vi "main OP600_V2 (AUTOMATISATION).vi"() -> ()   [LabVIEW 2020]
uses:
  Lib/02 SLIM ZEN WS 500/SubVi/FGV.ctl
  SubVI/CheminDeBase.vi
  SubVI/OP500ZP_state.ctl
  VG/VG_progressBar.vi
  VG/IS30%.vi
  VG/PN.vi
  VG/PackType.vi
  SubVI/OP500ZP_VGConf.vi
  VG/Ubatt.vi
panel:
  out "IS30% ?":bool
  out "Cluster":T1
  out "VISA OUT":T2
  out "progression":u8(slide) scale=0.0..100.0
  out "PN":string
  out "errout 2":errorcluster={"status"=TRUE, "code"=0, "source"="PCAN_CHANNEL ILLEGAL"} caption="errout"
  out "errout":errorcluster caption="sortie d'erreur"
  out "STOP":bool
  out "TOP":string
  out "DRAW":picture
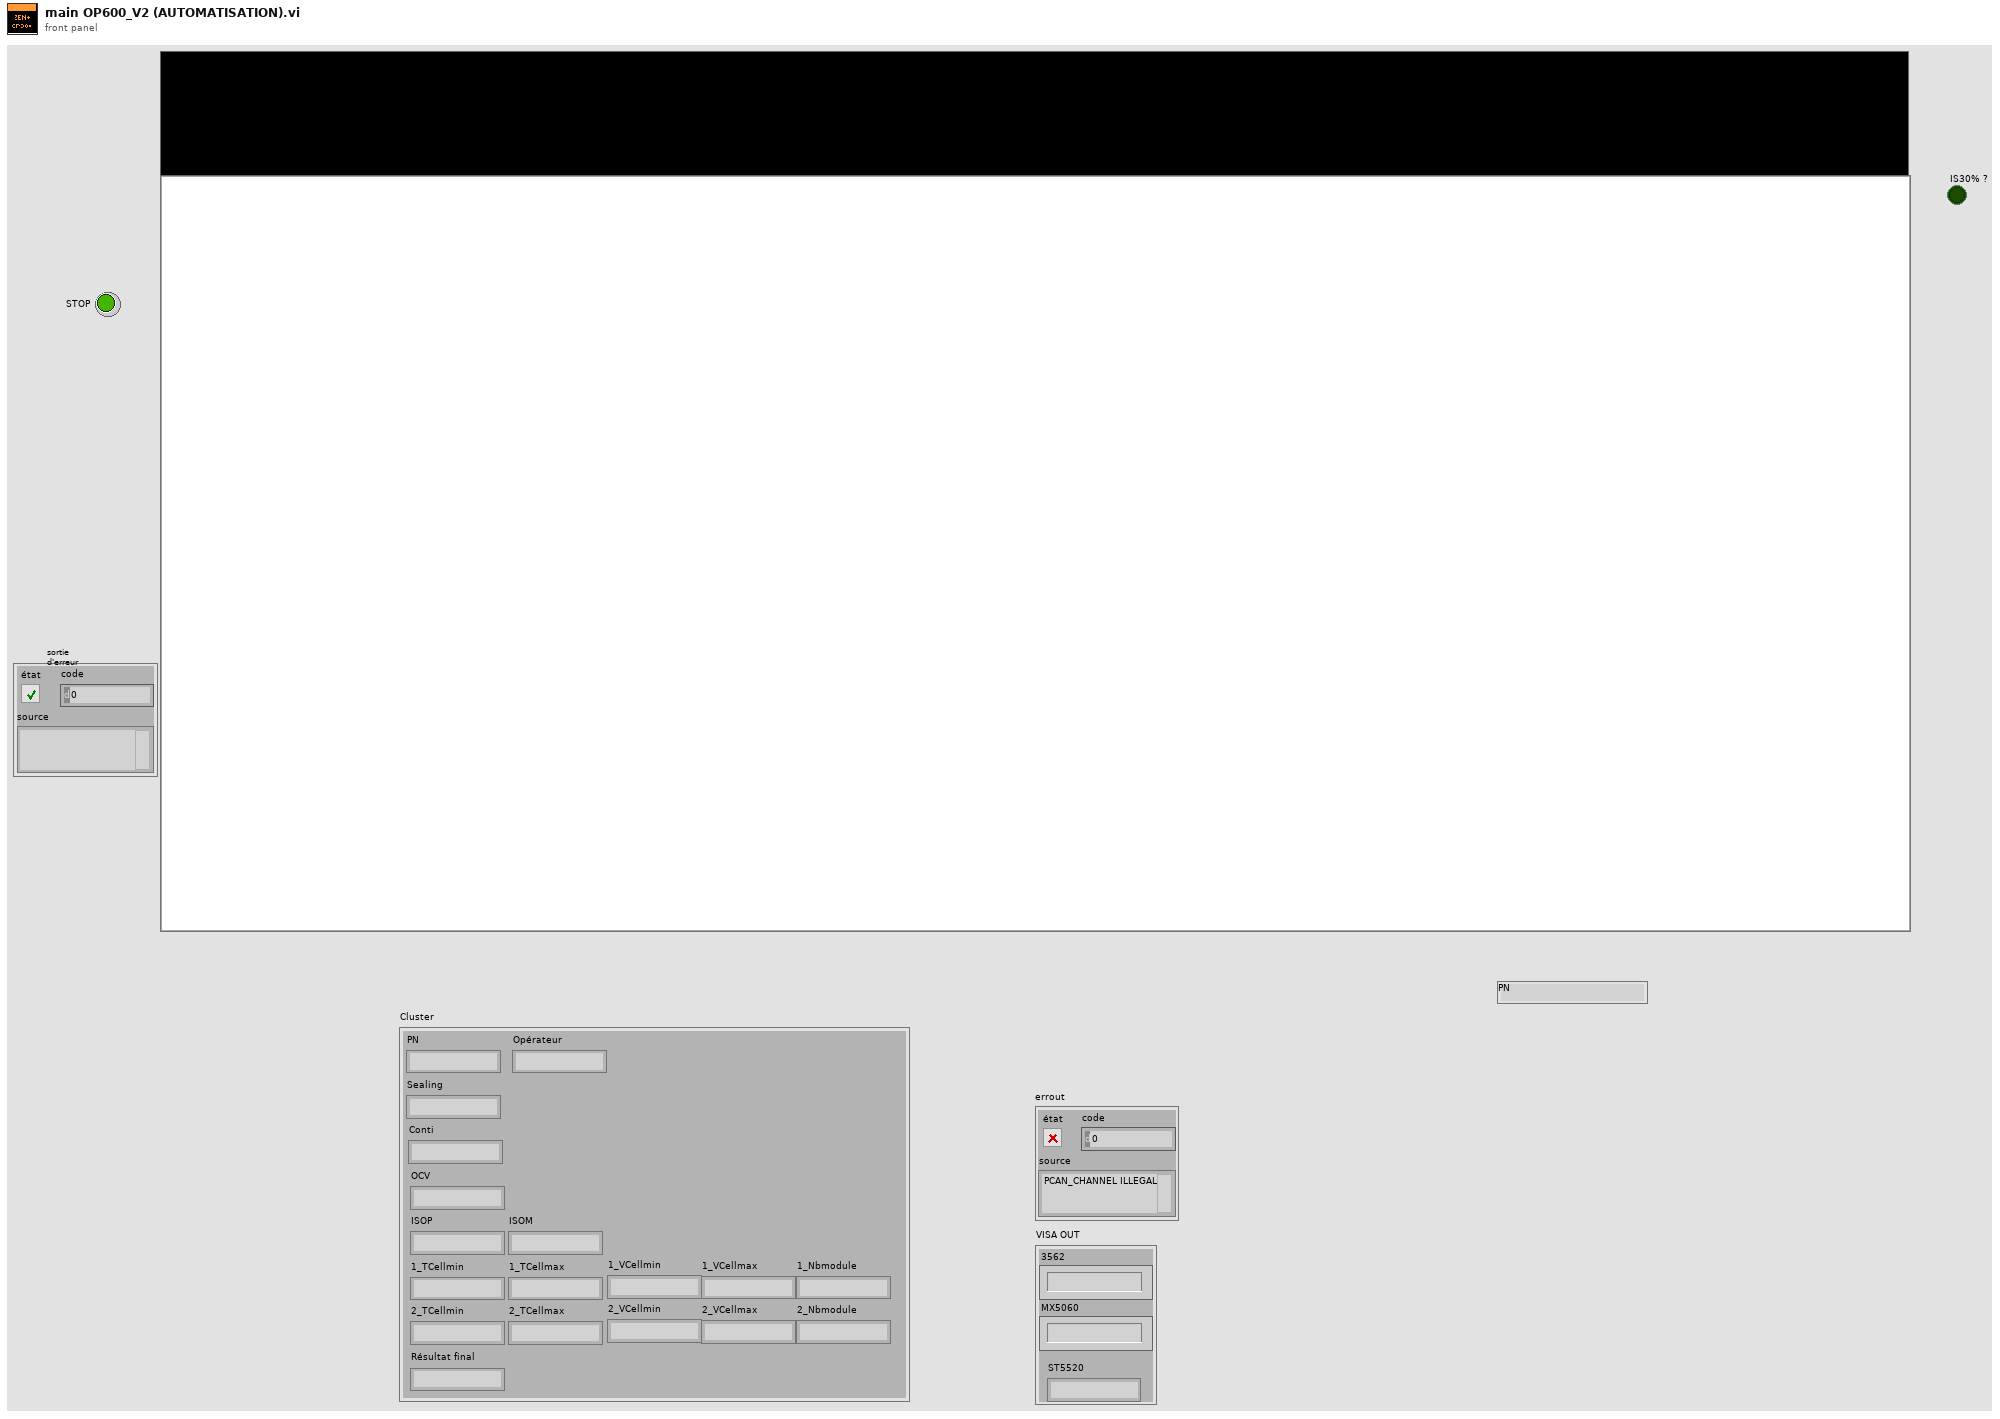
[diagram p1: front panel]
types:
  T1 = cluster{"PN":string, "Opérateur":string, "Sealing":string, "Conti":string, "OCV":string, "ISOP":string, "ISOM":string, "1_TCellmin":string, "1_TCellmax":string, "1_VCellmin":string, "1_VCellmax":string, "1_Nbmodule":string, "2_TCellmin":string, "2_TCellmax":string, "2_VCellmin":string, "2_VCellmax":string, "2_Nbmodule":string, "Résultat final":string}
  T2 = cluster{"3562":string, "MX5060":string, "ST5520":string}
  T3 = cluster{"PN":string, "Sealing":string, "Opérateur":string, "Conti":string, "OCV":string, "ISOP":string, "ISOM":string, "1_TCellmin":string, "1_TCellmax":string, "1_VCellmin":string, "1_VCellmax":string, "1_Nbmodule":string, "2_TCellmin":string, "2_TCellmax":string, "2_VCellmin":string, "2_VCellmax":string, "2_Nbmodule":string, "Résultat final":string}
  T4 = typedef "OP500ZP_state.ctl" = enum16{"Null", "Demarrage", "Init", "Scan", "Iso", "Softs", "MCU", "OCVACIR", "Conti", "DTC", "DataDyn", "DataDyn2", "Crash", "Next", "Comext"}
  T5 = typedef "FGV.ctl" = enum16{"GET", "SET", "RAZ"}
  T6 = typedef "OP500ZP_state.ctl" = enum16{"Null", "Demarrage", "Init", "Scan", "Montage", "Conti", "OCV", "Iso", "Softs", "Vpack", "DataDyn", "Dessouter", "DataDyn2", "Demontage", "Crash", "Next", "Sealing", "Comext"}
  T7 = cluster{"Chaîne":string, "Chaîne":string, "Chaîne":string, "Chaîne":string, "Chaîne":string, "Chaîne":string, "Chaîne":string, "Chaîne 2":string}
  T8 = typedef "imagedata.ctl" = cluster{"image type":i32, "image depth":i32, "image":u8[], "mask":u8[], "colors":u32[], "Rectangle":cluster{"left":i16, "top":i16, "right":i16, "bottom":i16}}
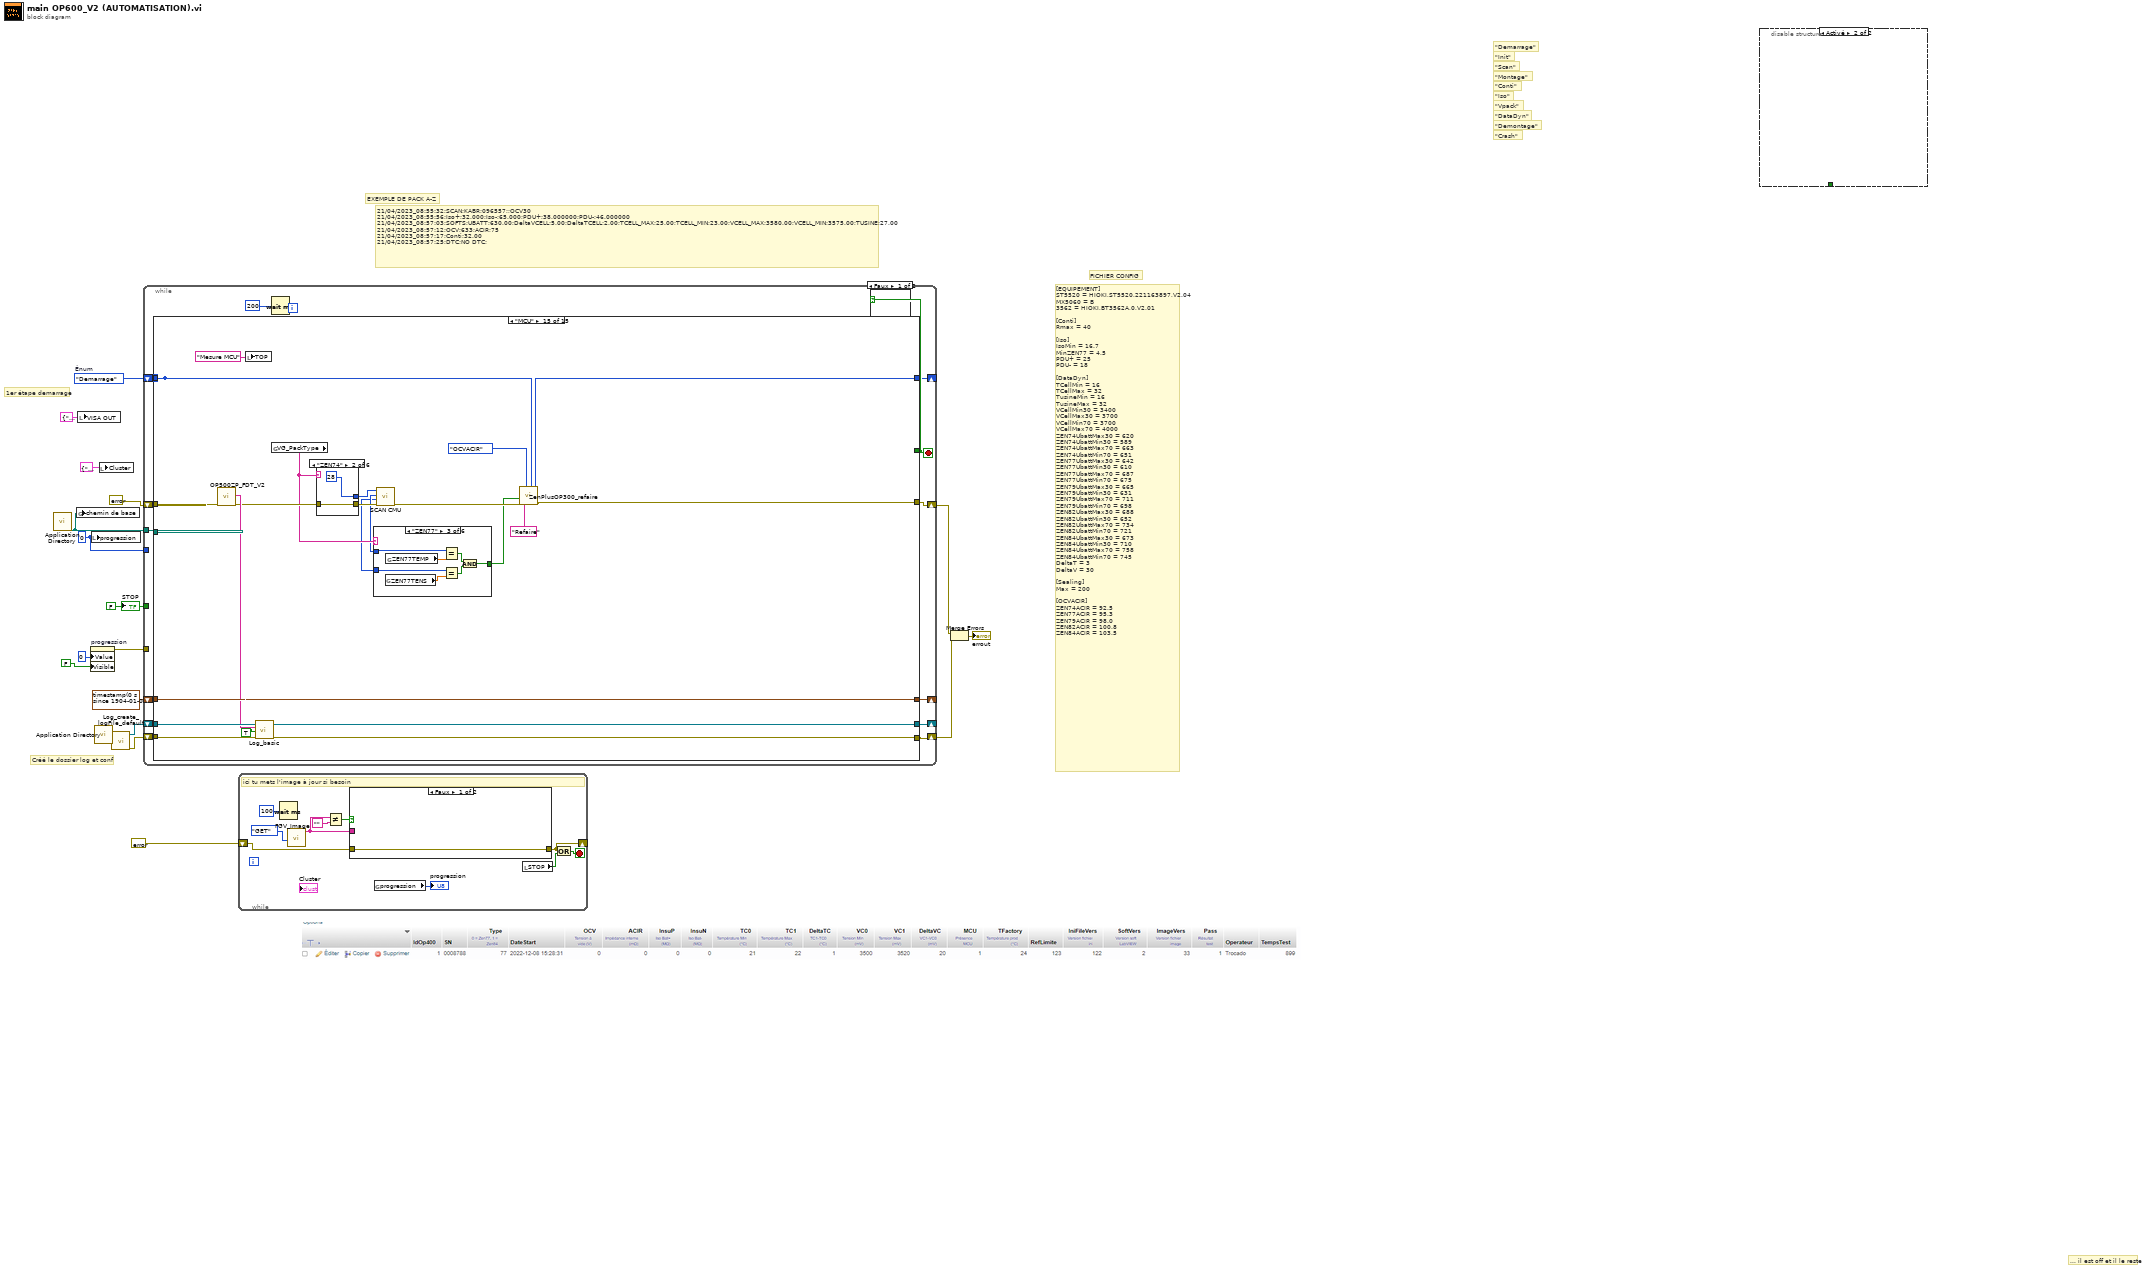
[diagram p0: block diagram]
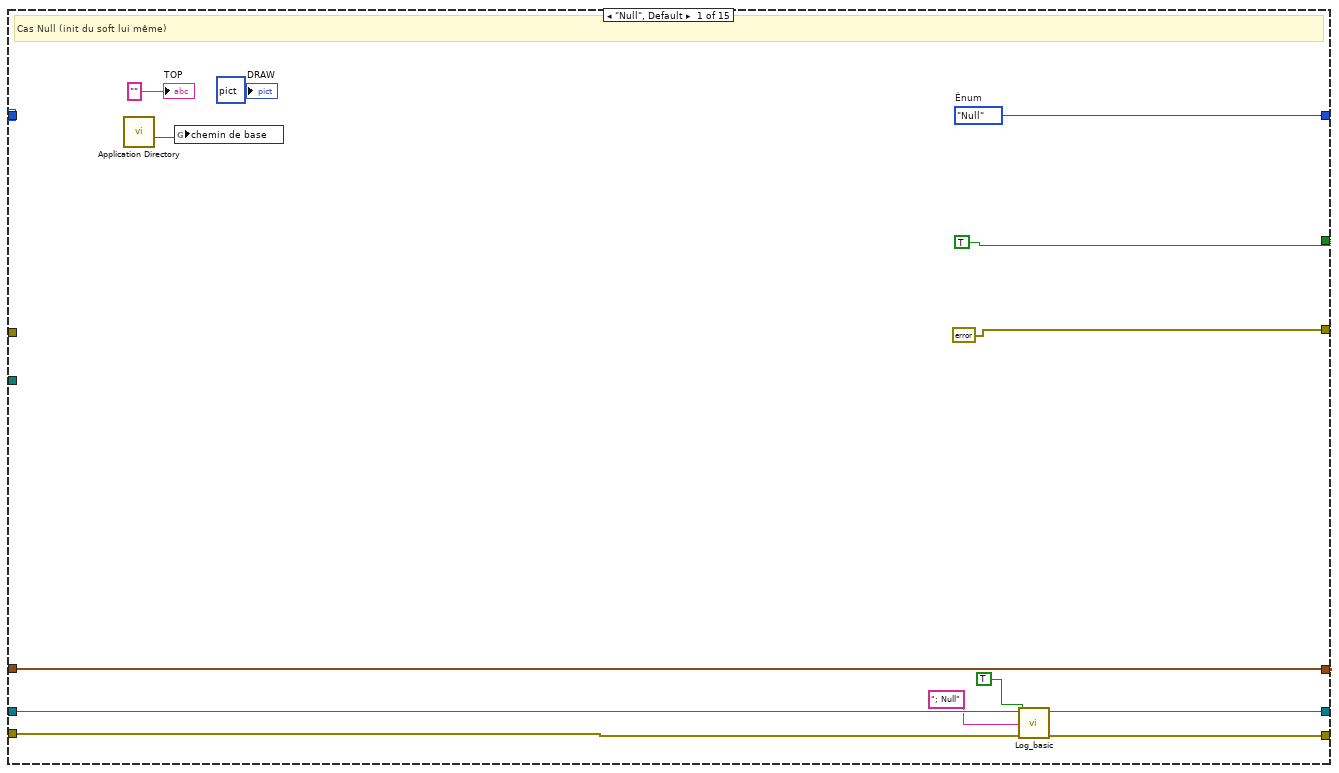
[diagram p2: hidden frame]
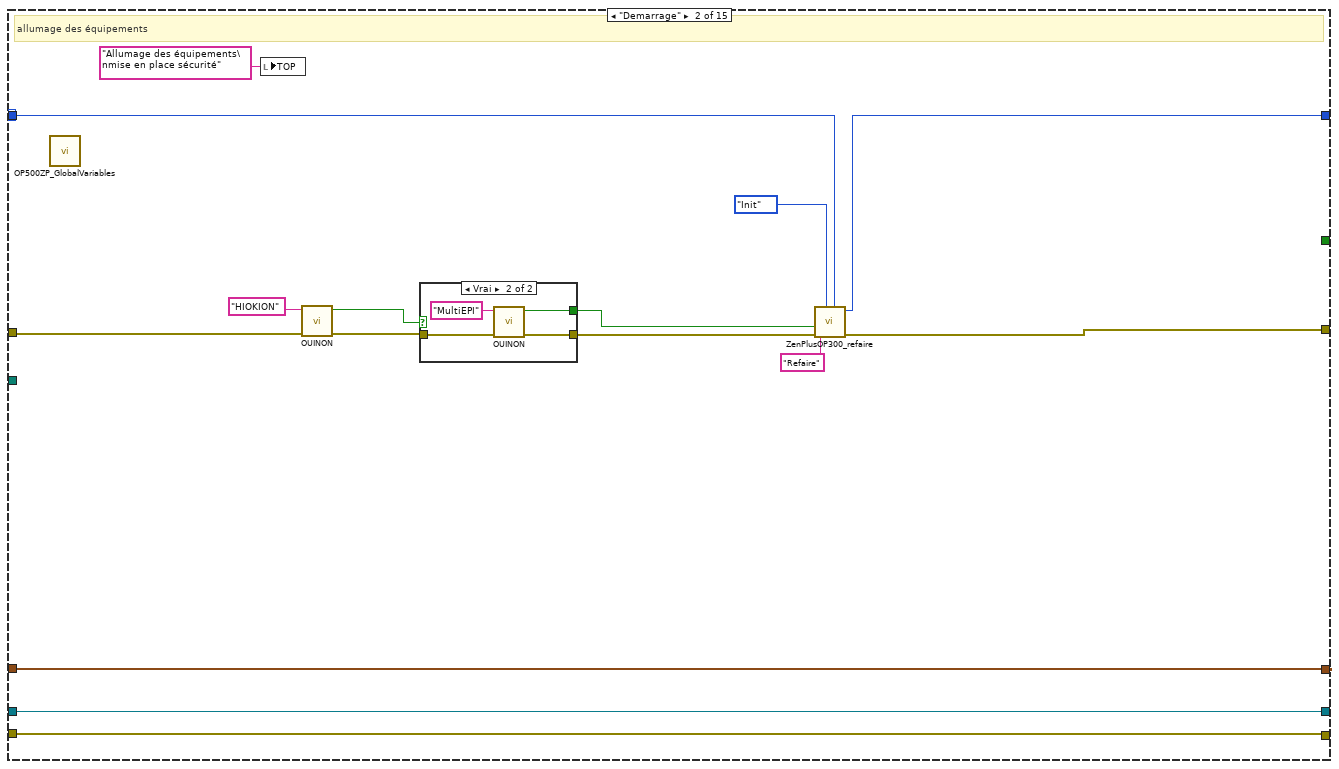
[diagram p3: hidden frame]
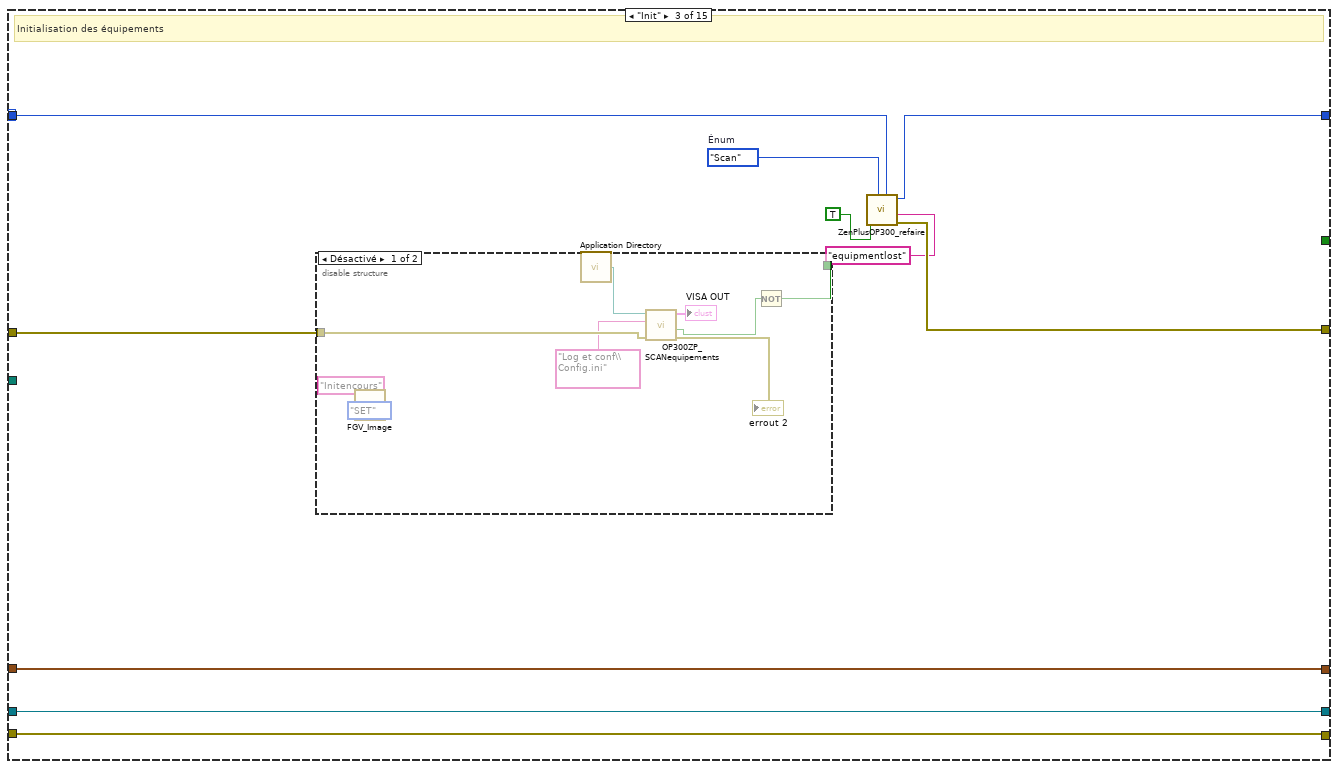
[diagram p5: hidden frame]
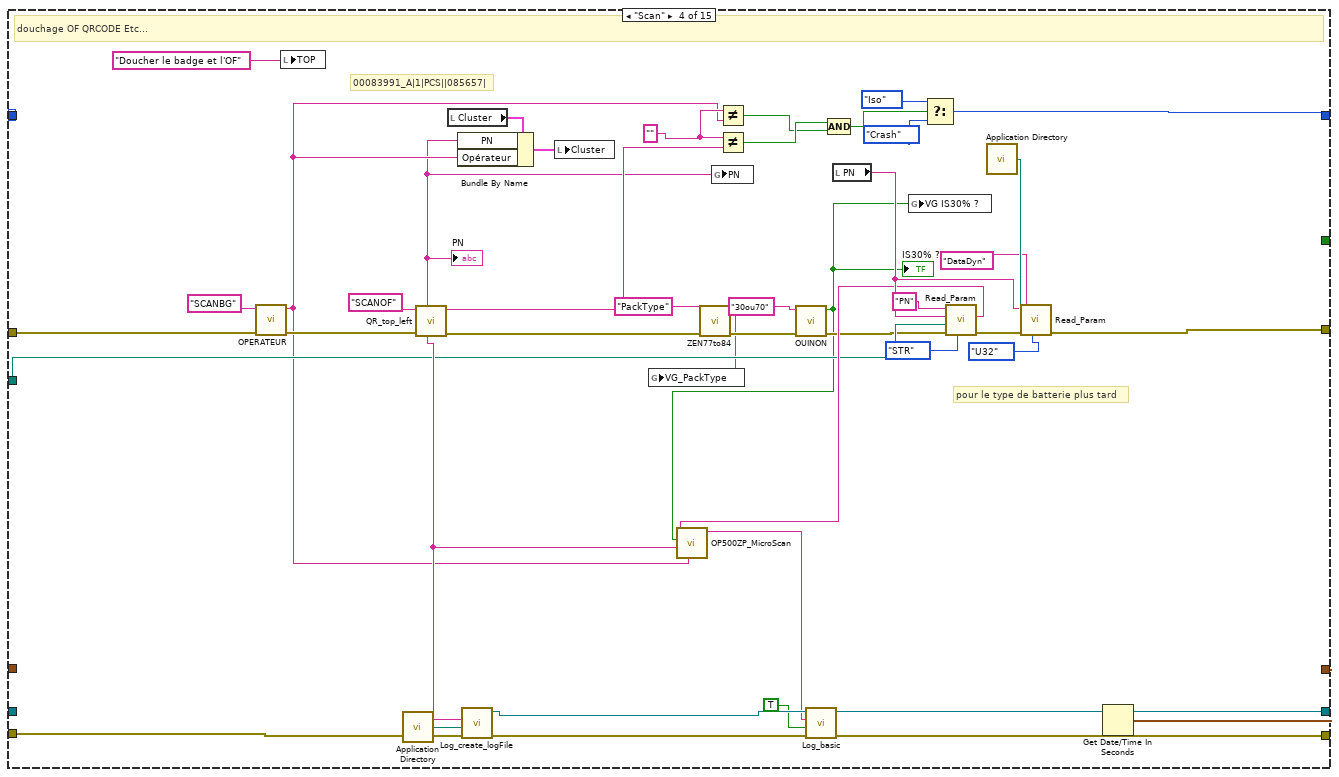
[diagram p7: hidden frame]
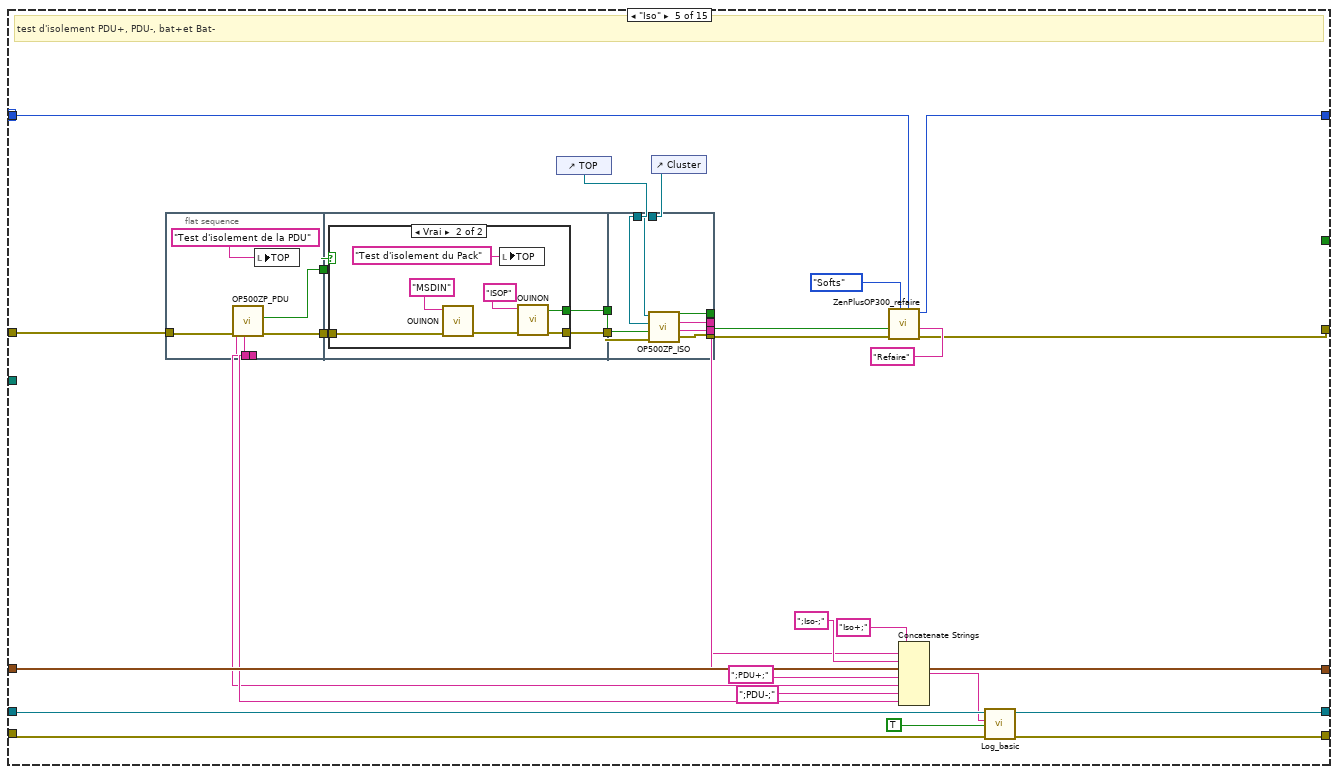
[diagram p8: hidden frame]
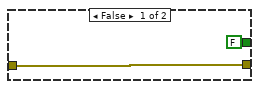
[diagram p9: hidden frame]
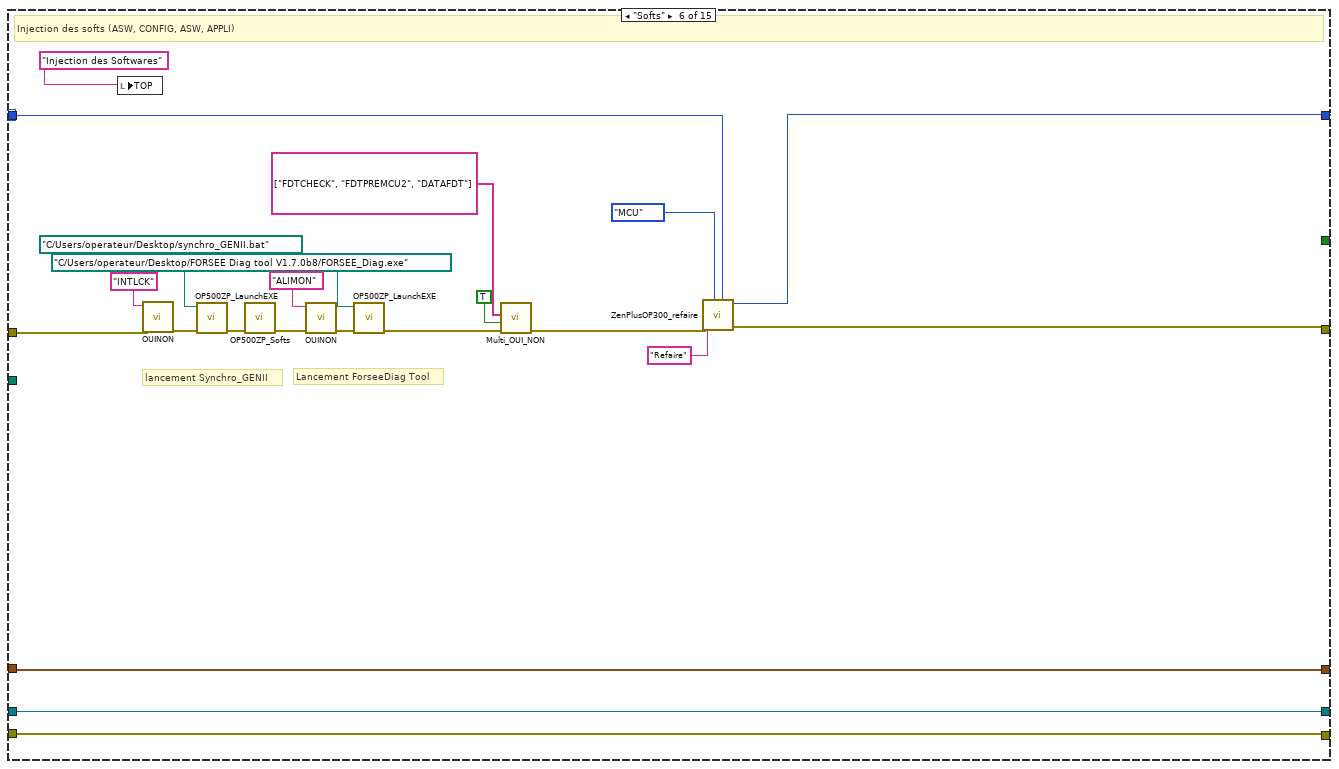
[diagram p10: hidden frame]
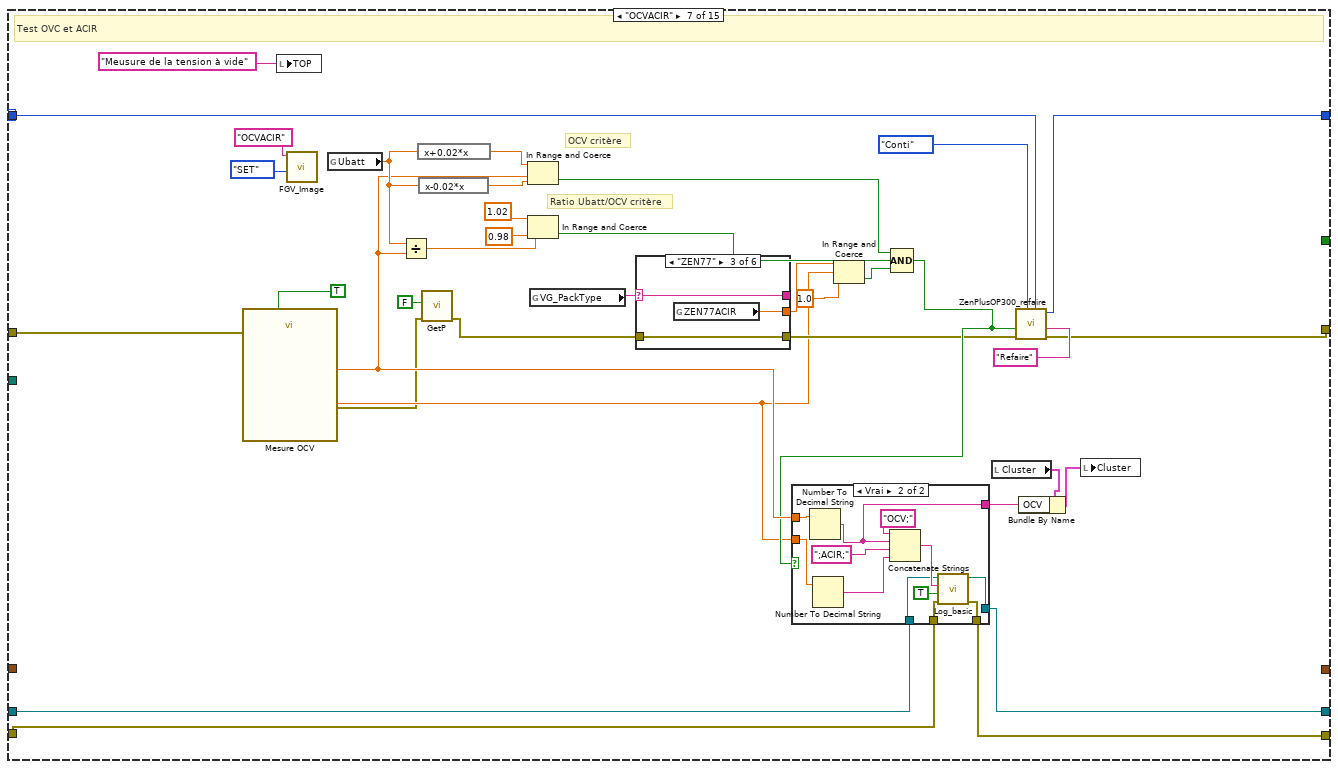
[diagram p11: hidden frame]
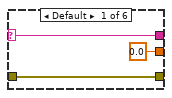
[diagram p12: hidden frame]
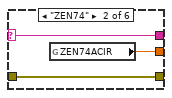
[diagram p13: hidden frame]
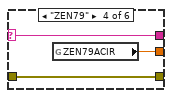
[diagram p14: hidden frame]
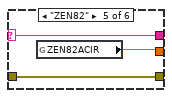
[diagram p15: hidden frame]
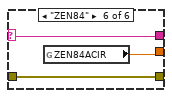
[diagram p16: hidden frame]
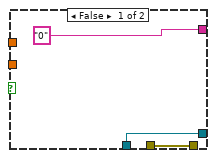
[diagram p17: hidden frame]
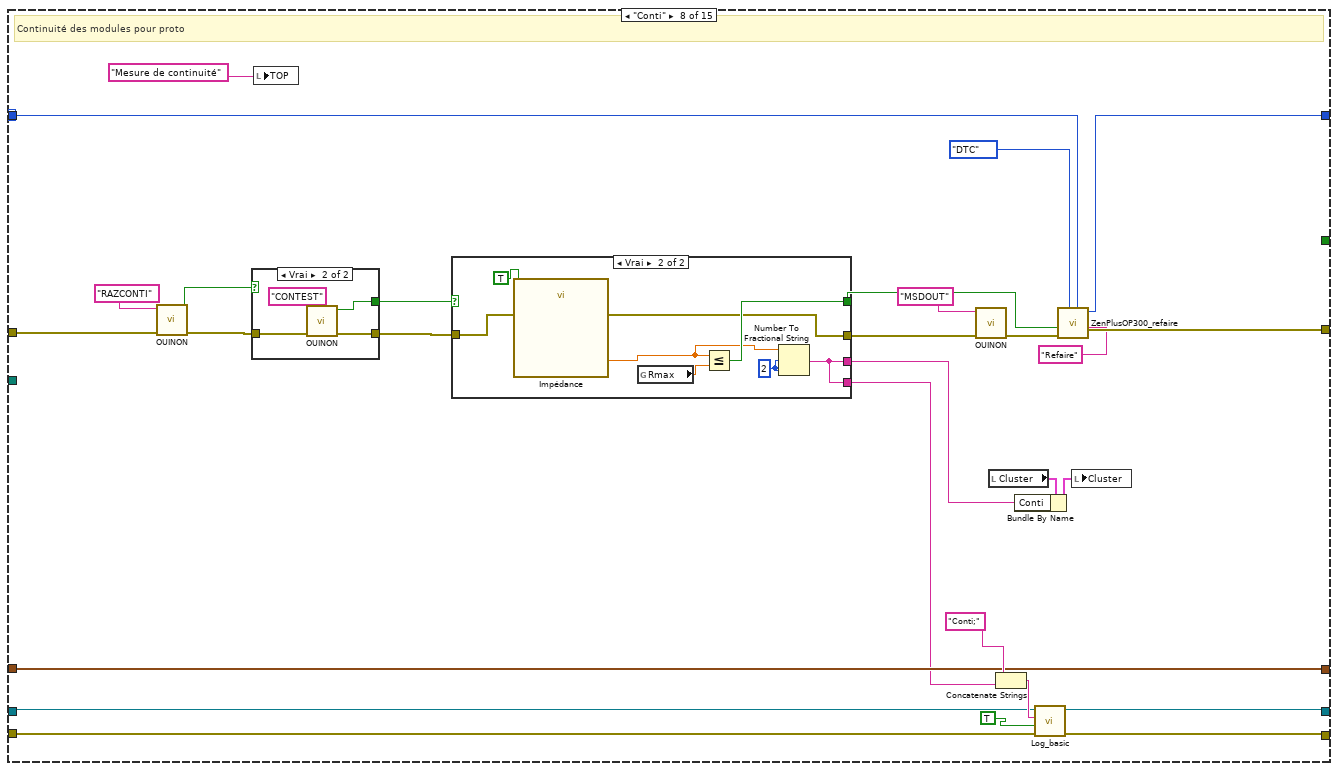
[diagram p18: hidden frame]
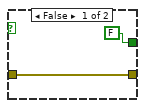
[diagram p19: hidden frame]
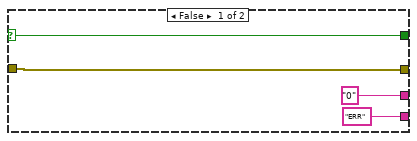
[diagram p20: hidden frame]
diagram:
  w8 = u8 0 ("progression")
  w1 = OP500ZP_state."Demarrage"  # Énum
  w14 = FALSE ("STOP")
  # "EXEMPLE DE PACK A-Z"
  # "21/04/2023_08:55:32;SCAN;KABR;096557;;OCV30\n21/04/2023_08:55:56;Iso+;32.000;Iso-;65.000;PDU+;38.000000;PDU-;46.000000\n21/04/2023_08:57:03;SOFTS;UBATT;630.00;DeltaVCELL;5.00;DeltaTCELL;2.00;TCELL_MAX;25.00;TCELL_MIN;23.00;VCELL_MAX;3580.00;VCELL_MIN;3575.00;TUSINE;27.00\n21/04/2023_08:57:12;OCV;633;ACIR;75\n21/04/2023_08:57:17;Conti;32.00\n21/04/2023_08:57:25;DTC;NO DTC;"
  # "FICHIER CONFIG"
  # "[EQUIPEMENT]\nST5520 = HIOKI,ST5520,221163897,V2.04\t\nMX5060 = B\n3562 = HIOKI,BT3562A,0,V2.01\n\n[Conti]\nRmax = 40\n\n[Iso]\nIsoMin = 16.7\nMinZEN77 = 4.5\nPDU+ = 25\nPDU- = 18\n\n[DataDyn]\nTCellMin = 16\nTCellMax = 32\nTusineMin = 16\nTusineMax = 32\nVCellMin30 = 3400\nVCellMax30 = 3700\nVCellMin70 = 3700\nVCellMax70 = 4000\nZEN74UbattMax30 = 620\nZEN74UbattMin30 = 589\nZEN74UbattMax70 = 663\nZEN74UbattMin70 = 651\nZEN77UbattMax30 = 642\nZEN77UbattMin30 = 610\nZEN77UbattMax70 = 687\nZEN77UbattMin70 = 675\nZEN79UbattMax30 = 665\nZEN79UbattMin30 = 631\nZEN79UbattMax70 = 711\nZEN79UbattMin70 = 698\nZEN82UbattMax30 = 688\nZEN82UbattMin30 = 652\nZEN82UbattMax70 = 734\nZEN82UbattMin70 = 721\nZEN84UbattMax30 = 673\nZEN84UbattMin30 = 710\nZEN84UbattMax70 = 758\nZEN84UbattMin70 = 745\nDeltaT = 3\nDeltaV = 30\n\n[Sealing]\nMax = 200\n\n[OCVACIR]\nZEN74ACIR = 92.5\nZEN77ACIR = 95.3\nZEN79ACIR = 98.0\nZEN82ACIR = 100.8\nZEN84ACIR = 103.5"
  # "Créé le dossier log et conf"
  # "1er étape demarrage"
  # "\"Crash\""
  # "\"Demontage\""
  # "\"DataDyn\""
  # "\"Iso\""
  # "\"Montage\""
  # "\"Scan\""
  # "\"Init\""
  # "\"Demarrage\""
  # "\"Conti\""
  # "\"Vpack\""
  # "... il est off et il le reste"
  n1 = call <vilib>:"Application Directory.vi"() -> ("Application Directory"=w13:path)
  n2 = global write "CheminDeBase.vi" "chemin de base"(w13) -> ()
  n3 = local write "VISA OUT"(T2 {"3562"="", "MX5060"="", "ST5520"=""} ("VISA OUT")) -> ()
  n4 = property on="progression" class="Gliss (strict)"("Value"=u8 0 ("progression"), "Visible"=FALSE) -> (error out=w6:errorcluster)  [unwired: 2 in, 1 out]
  n5 = local write "progression"(w8) -> ()
  n6 = call <vilib>:"Application Directory.vi"() -> ("Application Directory"=w11:path)
  n7 = local write "Cluster"(T3 {"PN"="0", "Sealing"="0", "Opérateur"="0", "Conti"="0", "OCV"="0", "ISOP"="0", "ISOM"="0", "1_TCellmin"="0", "1_TCellmax"="0", "1_VCellmin"="0", "1_VCellmax"="0", "1_Nbmodule"="0", "2_TCellmin"="0", "2_TCellmax"="0", "2_VCellmin"="0", "2_VCellmax"="0", "2_Nbmodule"="0", "Résultat final"="0"} ("Cluster")) -> ()
  n8 = call "Log_create_logFile_default.vi"("appdir"=w11) -> ("errout"=w12:errorcluster, "Fichier à flux d'octets en sortie"=w15:refnum<file>)  [unwired: 9 in]
  n9 = while {
    shift-right: [w30] -> w17
    shift-left: errorcluster {"status"=FALSE, "code"=0, "source"=""} ("error out") -> [w21]
    shift-right: [w26] -> w16
    shift-left: w12 -> [w29]
    shift-right: [w27] -> _
    shift-left: w15 -> [w28]
    tunnel: w13 -> [w24]
    tunnel: w14 -> [_]
    shift-right: [w22] -> _
    shift-left: timestamp(0 s since 1904-01-01) ("seconds since 1Jan1904") -> [w23]
    tunnel: w8 -> [_]
    tunnel: w6 -> [_]
    shift-right: [w20] -> _
    shift-left: w1 -> [w19]
    stop <- w25 stop-if-true
    n10 = case shown="\"MCU\"" w19 {
      selector: w19 -> [_ w48 w70 _ _ w188 w234 w291 w341 _ w419 _ _ w541 w610]
      tunnel: w21 -> [_ w58 w72 w128 w138 w197 w233 w303 w328 w389 w411 w495 w532 w538 w617]
      tunnel: [errorcluster {"status"=FALSE, "code"=0, "source"=""} ("errin") w49 w71 w108 w133 w190 w232 w292 w342 w393 w412 w495 w504 w540 w612] -> w30
      tunnel: w29 -> [w40 w52 w75 w124 w155 w202 w229 w299 w334 w398 w415 w498 w529 w544 w621]
      tunnel: w28 -> [w41 w59 w74 _ w154 w201 w231 w298 w332 w397 w417 w499 w530 w543 w620]
      tunnel: [w38 w59 w74 w126 w153 w201 w230 w297 w331 w396 w413 _ _ w535 w618] -> w27
      tunnel: [w39 w52 w75 w127 w156 w202 w228 w296 w333 w395 w414 w471 w502 w542 w619] -> w26
      tunnel: [TRUE _ _ _ _ _ _ _ _ _ _ w500 _ _ _] -> w25
      tunnel: w24 -> [_ _ _ w102 _ _ _ _ _ _ w418 _ _ w539 _]
      tunnel: w23 -> [w35 w57 w73 _ w152 w206 _ w294 w329 w376 w416 _ _ w536 w616]
      tunnel: [w35 w57 w73 w116 w152 w206 _ w294 w329 w376 w416 _ _ w537 w616] -> w22
      tunnel: [w32 w46 w68 w85 w130 w189 w216 w280 w339 w374 w410 OP500ZP_state."Crash" w503 w534 w609] -> w20
      tunnel: w19 -> [_ _ _ _ w131 _ _ _ _ _ _ _ _ _ _]
      frame "Null", Default {
        w32 = OP500ZP_state."Null"  # Énum
        # "Cas Null (init du soft lui même)"
        n11 = call <vilib>:"Application Directory.vi"() -> ("Application Directory"=w44:path)
        n12 = global write "CheminDeBase.vi" "chemin de base"(w44) -> ()
        n13 = call "Log_basic.vi"("errin"=w40, "date?"=TRUE, "chaîne"="; Null", "in"=w41) -> ("sortie d'erreur"=w39:errorcluster, "refnum en sortie"=w38:refnum<file>)  [unwired: 6 in]
        "DRAW" <- picture data[5B] ("DRAW")
        "TOP" <- "" ("TOP")
      }
      frame "Demarrage" {
        # "allumage des équipements"
        n14 = call "OP500ZP_GlobalVariables.vi"() -> ()  [unwired: 12 in]
        n15 = local write "TOP"("Allumage des équipements\nmise en place sécurité" ("TOP")) -> ()
        n16 = call "OUINON.vi"("errin"=w58, "image"="HIOKION") -> ("error out"=w53:errorcluster, "OUI/NON"=w54:bool)  [unwired: 8 in]
        n17 = case shown="Vrai" w54 {
          selector: w54 -> [w61 _]
          tunnel: [w61 w65] -> w45
          tunnel: [w60 w64] -> w50
          tunnel: w53 -> [w60 w62]
          frame False {
          }
          frame True {
            n18 = call "OUINON.vi"("errin"=w62, "image"="MultiEPI" ("IN")) -> ("error out"=w64:errorcluster, "OUI/NON"=w65:bool)  [unwired: 8 in]
          }
        }
        n19 = call "ZenPlusOP300_refaire.vi"("image"="Refaire", "refaire"=w48, "casOK"=OP500ZP_state."Init", "errin"=w50, "test ok ?"=w45) -> ("errout"=w49:errorcluster, "Next"=w46:T4)  [unwired: 5 in]
      }
      frame "Init" {
        w67 = OP500ZP_state."Scan"  # Énum
        # "Initialisation des équipements"
        n20 = disable-structure shown="Désactivé" {
          disable-tunnel: w72 -> [w84 _]
          disable-tunnel: [w79 _] -> _
          frame Disabled {
            n21 = call "FGV_Image.vi"("Énum"=FGV."SET", "IN"="Initencours") -> ()  [unwired: 9 in, 1 out]
            n22 = call <vilib>:"Application Directory.vi"() -> ("Application Directory"=w80:path)
            n23 = call "OP300ZP_SCANequipements.vi"("Errin"=w84, "Chaîne"="Log et conf\\Config.ini", "pathin"=w80) -> ("errout"=→"errout 2":errorcluster, "KO?"=w78:bool, "VISA OUT"=→"VISA OUT":T2)  [unwired: 6 in]
            n24 = Not(x=w78) -> (.not. x?=w79:bool)
          }
          frame Enabled {
          }
        }
        n25 = call "ZenPlusOP300_refaire.vi"("image"="equipmentlost", "refaire"=w70, "casOK"=w67, "test ok ?"=TRUE) -> ("errout"=w71:errorcluster, "Next"=w68:T4)  [unwired: 6 in]
      }
      frame "Scan" {
        w119 = "" ("x")
        # "pour le type de batterie plus tard"
        # "00083991_A|1|PCS||085657|"
        # "douchage OF QRCODE Etc..."
        n26 = call "OPERATEUR.vi"("errin"=w128, "IN"="SCANBG") -> ("error out"=w115:errorcluster, "Dataout"=w94:string)  [unwired: 8 in]
        n27 = local write "TOP"("Doucher le badge et l'OF" ("TOP")) -> ()
        n28 = call <vilib>:"Application Directory.vi"() -> ("Application Directory"=w125:path)
        n29 = call "QR_top_left.vi"("errin"=w115, "image"="SCANOF") -> ("error out"=w89:errorcluster, "Réponse"=w113:string, "SN"=w112:string, "PN"=w90:string)  [unwired: 5 in, 1 out]
        "PN" <- w90
        n30 = local read "Cluster"() -> (w96:T1)
        n31 = Bundle By Name(cluster=w96, "PN"=w90, "Opérateur"=w94) -> (w95:T1)
        n32 = call "Log_create_logFile.vi"("errin"=w124, "toute l'expression"=w112, "Application Directory"=w125) -> ("sortie d'erreur"=w122:errorcluster, "Fichier à flux d'octets en sortie"=w123:refnum<file>)  [unwired: 7 in]
        n33 = local write "Cluster"(w95) -> ()
        n34 = call "ZEN77to84.vi"("errin"=w89, "image"="PackType") -> ("error out"=w88:errorcluster, "Réponse"=w86:string)  [unwired: 8 in]
        n35 = global write "PackType.vi" "VG_PackType"(w86) -> ()
        n36 = global write "PN.vi" "PN"(w90) -> ()
        n37 = Not Equal?(x=w119, y=w94) -> (x != y?=w117:bool)
        n38 = Not Equal?(x=w119, y=w113) -> (x != y?=w118:bool)
        n39 = call "OUINON.vi"("errin"=w88, "image"="30ou70") -> ("error out"=w92:errorcluster, "OUI/NON"=w91:bool)  [unwired: 8 in]
        "IS30% ?" <- w91
        n40 = Compound Arithmetic op=AND ("Opérateur arithmétique")(w118, w117) -> (w100:bool)
        n41 = local read "PN"() -> (w104:string)
        n42 = global write "IS30%.vi" "VG IS30% ?"(w91) -> ()
        n43 = Select ("Sélectionner")(t=OP500ZP_state."Iso" ("Énum"), s=w100, f=OP500ZP_state."Crash" ("cas faux")) -> (s? t:f=w85:T4)
        n44 = call "Read_Param.vi"("Énum"=enum16{"STR", "DBL", "U32"}."STR", "errin"=w92, "pathin"=w102, "section"=w104, "key"="PN") -> ("error out"=w107:errorcluster, "str"=w103:string)  [unwired: 2 in, 3 out]
        n45 = call "OP500ZP_MicroScan.vi"("Dataout"=w94, "SN"=w112, "Oui"=w91, "str"=w103) -> ("Chaîne"=w121:string)  [unwired: 7 in]
        n46 = call "Log_basic.vi"("errin"=w122, "date?"=TRUE, "chaîne"=w121, "in"=w123) -> ("sortie d'erreur"=w127:errorcluster, "refnum en sortie"=w126:refnum<file>)  [unwired: 6 in]
        n47 = call <vilib>:"Application Directory.vi"() -> ("Application Directory"=w111:path)
        n48 = call "Read_Param.vi"("Énum"=enum16{"STR", "DBL", "U32"}."U32", "errin"=w107, "pathin"=w111, "section"="DataDyn", "key"=w104) -> ("error out"=w108:errorcluster)  [unwired: 2 in, 4 out]
        n49 = Get Date/Time In Seconds() -> (seconds since 1Jan1904=w116:timestamp)
      }
      frame "Iso" {
        # "test d'isolement PDU+, PDU-, bat+et Bat-"
        n50 = flat-sequence {
          tunnel: [w161] -> w140
          tunnel: [w162] -> w139
          tunnel: w138 -> [w163]
          tunnel: [w160] -> w137
          tunnel: [w159] -> w136
          tunnel: [w165] -> w142
          tunnel: [w164] -> w141
          tunnel: w140 -> [w167]
          tunnel: w139 -> [w166]
          tunnel: [w184] -> w134
          tunnel: [w183] -> w149
          tunnel: [w182] -> w147
          tunnel: w144 -> [w179]
          tunnel: w143 -> [w178]
          tunnel: w142 -> [w181]
          tunnel: w141 -> [w180]
          tunnel: [w177] -> w129
          frame #0 {
            n51 = call "OP500ZP_PDU.vi"("errin"=w163) -> ("errout"=w162:errorcluster, "PASS?"=w161:bool, "ISO_PDU-"=w160:string, "ISO_PDU+"=w159:string)  [unwired: 7 in]
            n52 = local write "TOP"("Test d'isolement de la PDU" ("TOP")) -> ()
          }
          frame #1 {
            n53 = case shown="Vrai" w167 {
              tunnel: w166 -> [w169 w173]
              tunnel: [w169 w175] -> w165
              tunnel: [FALSE ("Oui") w174] -> w164
              frame False {
              }
              frame True {
                n54 = call "OUINON.vi"("errin"=w173, "image"="MSDIN") -> ("error out"=w172:errorcluster)  [unwired: 8 in, 1 out]
                n55 = local write "TOP"("Test d'isolement du Pack" ("TOP")) -> ()
                n56 = call "OUINON.vi"("errin"=w172, "image"="ISOP" ("IN")) -> ("error out"=w175:errorcluster, "OUI/NON"=w174:bool)  [unwired: 8 in]
              }
            }
          }
          frame #2 {
            n57 = call "OP500ZP_ISO.vi"("entrée d'erreur (pas d'erreur)"=w181, "Oui"=w180, "reference en entrée"=w178, "Cluster en entrée"=w179) -> ("sortie d'erreur"=w184:errorcluster, "Chaîne 2"=w183:string, "Chaîne"=w182:string, "Booléen"=w177:bool)  [unwired: 4 in]
          }
        }
        n58 = control-ref of="TOP"() -> (w143:refnum<vi>)
        n59 = control-ref of="Cluster"() -> (w144:refnum<vi>)
        n60 = call "ZenPlusOP300_refaire.vi"("image"="Refaire", "refaire"=w131, "casOK"=OP500ZP_state."Softs", "errin"=w134, "test ok ?"=w129) -> ("errout"=w133:errorcluster, "Next"=w130:T4)  [unwired: 5 in]
        n61 = Concatenate Strings("Iso+;" ("chaîne"), w147, ";Iso-;" ("chaîne"), w149, ";PDU+;" ("chaîne"), w136, ";PDU-;" ("chaîne"), w137) -> (w148:string)
        n62 = call "Log_basic.vi"("errin"=w155, "date?"=TRUE, "chaîne"=w148, "in"=w154) -> ("sortie d'erreur"=w156:errorcluster, "refnum en sortie"=w153:refnum<file>)  [unwired: 6 in]
      }
      frame "Softs" {
        # "Lancement ForseeDiag Tool"
        # "lancement Synchro_GENII"
        # "Injection des softs (ASW, CONFIG, ASW, APPLI)"
        n63 = local write "TOP"("Injection des Softwares" ("TOP")) -> ()
        n64 = call "OUINON.vi"("errin"=w197, "image"="INTLCK") -> ("error out"=w196:errorcluster)  [unwired: 8 in, 1 out]
        n65 = call "OP500ZP_LaunchEXE.vi"("errin"=w196, "Application à lancer"=path "C:/Users/operateur/Desktop/synchro_GENII.bat") -> ("error out"=w205:errorcluster)  [unwired: 7 in]
        n66 = call "OP500ZP_Softs.vi"("errin"=w205) -> ("errout"=w194:errorcluster)  [unwired: 9 in, 1 out]
        n67 = call "OUINON.vi"("errin"=w194, "image"="ALIMON") -> ("error out"=w193:errorcluster)  [unwired: 8 in, 1 out]
        n68 = call "OP500ZP_LaunchEXE.vi"("errin"=w193, "Application à lancer"=path "C:/Users/operateur/Desktop/FORSEE Diag tool V1.7.0b8/FORSEE_Diag.exe") -> ("error out"=w200:errorcluster)  [unwired: 7 in]
        n69 = call "Multi_OUI_NON.vi"("errin"=w200, "errinb"=TRUE, "Tableau"=string[] ["FDTCHECK", "FDTPREMCU2", "DATAFDT"]) -> ("errout"=w191:errorcluster)  [unwired: 7 in, 1 out]
        n70 = call "ZenPlusOP300_refaire.vi"("image"="Refaire", "refaire"=w188, "casOK"=OP500ZP_state."MCU", "errin"=w191) -> ("errout"=w190:errorcluster, "Next"=w189:T4)  [unwired: 6 in]
      }
      frame "OCVACIR" {
        # "Ratio Ubatt/OCV critère"
        # "OCV critère"
        # "Test OVC et ACIR"
        n71 = call "Mesure OCV"("Enable"=TRUE, "error in (no error)"=w233) -> ("Résistance (Ohm)"=w210:dbl, "Tension Bat+ Bat- (V)"=w223:dbl, "error out"=w209:errorcluster)  [unwired: 14 in, 1 out]
        n72 = local write "TOP"("Meusure de la tension à vide" ("TOP")) -> ()
        n73 = call "FGV_Image.vi"("Énum"=FGV."SET", "IN"="OCVACIR") -> ()  [unwired: 9 in, 1 out]
        n74 = global read "Ubatt.vi" "Ubatt"() -> (w224:dbl)
        n75 = Divide(x=w224, y=w223) -> (x/y=w222:dbl)
        n76 = expression code="x+0.02*x"(w224) -> (w225:dbl)
        n77 = expression code="x-0.02*x"(w224) -> (w226:dbl)
        n78 = call "GetP.vi"("errin"=w209, "Pédale ON?"=FALSE) -> ("errout"=w208:errorcluster)  [unwired: 8 in, 1 out]
        n79 = In Range and Coerce(upper limit=w225, x=w223, lower limit=w226) -> (In Range?=w219:bool)  [unwired: 1 out]
        n80 = In Range and Coerce(upper limit=1.02 ("limite supérieure"), x=w222, lower limit=0.98 ("limite inférieure")) -> (In Range?=w218:bool)  [unwired: 1 out]
        n81 = global read "PackType.vi" "VG_PackType"() -> (w227:string)
        n82 = case shown="\"ZEN77\"" w227 {
          selector: w227 -> [w245 w248 w251 w254 w257 w260]
          tunnel: [w245 w248 w251 w254 w257 w260] -> _
          tunnel: [0.0 ("ZEN84ACIR") w247 w250 w253 w256 w259] -> w215
          tunnel: [w243 w246 w249 w252 w255 w258] -> w211
          tunnel: w208 -> [w243 w246 w249 w252 w255 w258]
          frame Default {
          }
          frame "ZEN74" {
            n83 = global read "OP500ZP_VGConf.vi" "ZEN74ACIR"() -> (w247:dbl)
          }
          frame "ZEN77" {
            n84 = global read "OP500ZP_VGConf.vi" "ZEN77ACIR"() -> (w250:dbl)
          }
          frame "ZEN79" {
            n85 = global read "OP500ZP_VGConf.vi" "ZEN79ACIR"() -> (w253:dbl)
          }
          frame "ZEN82" {
            n86 = global read "OP500ZP_VGConf.vi" "ZEN82ACIR"() -> (w256:dbl)
          }
          frame "ZEN84" {
            n87 = global read "OP500ZP_VGConf.vi" "ZEN84ACIR"() -> (w259:dbl)
          }
        }
        n88 = In Range and Coerce(upper limit=w215, x=w210, lower limit=1.0 ("limite inférieure")) -> (In Range?=w213:bool)  [unwired: 1 out]
        n89 = Compound Arithmetic op=AND ("Opérateur arithmétique")(w219, w218, w213) -> (w212:bool)
        n90 = case shown="Vrai" w212 {
          tunnel: [w261 w272] -> w230
          tunnel: w223 -> [_ w271]
          tunnel: ["0" w270] -> w235
          tunnel: w231 -> [w261 w269]
          tunnel: w229 -> [w262 w268]
          tunnel: [w262 w267] -> w228
          tunnel: w210 -> [_ w265]
          frame False {
          }
          frame True {
            n91 = Number To Decimal String(number=w271) -> (decimal integer string=w270:string)  [unwired: 1 in]
            n92 = Number To Decimal String(number=w265) -> (decimal integer string=w264:string)  [unwired: 1 in]
            n93 = Concatenate Strings("OCV;" ("chaîne"), w270, ";ACIR;" ("chaîne"), w264) -> (w274:string)
            n94 = call "Log_basic.vi"("errin"=w268, "date?"=TRUE, "chaîne"=w274, "in"=w269) -> ("sortie d'erreur"=w267:errorcluster, "refnum en sortie"=w272:refnum<file>)  [unwired: 6 in]
          }
        }
        n95 = local read "Cluster"() -> (w237:T1)
        n96 = call "ZenPlusOP300_refaire.vi"("image"="Refaire", "refaire"=w234, "casOK"=OP500ZP_state."Conti" ("Énum"), "errin"=w211, "test ok ?"=w212) -> ("errout"=w232:errorcluster, "Next"=w216:T4)  [unwired: 5 in]
        n97 = Bundle By Name(cluster=w237, "OCV"=w235) -> (w236:T1)
        n98 = local write "Cluster"(w236) -> ()
      }
      frame "Conti" {
        # "Continuité des modules pour proto"
        n99 = call "OUINON.vi"("errin"=w303, "image"="RAZCONTI" ("IN")) -> ("error out"=w285:errorcluster, "OUI/NON"=w283:bool)  [unwired: 8 in]
        n100 = case shown="Vrai" w283 {
          tunnel: w285 -> [w305 w309]
          tunnel: [w305 w308] -> w284
          tunnel: [FALSE ("Oui") w307] -> w282
          frame False {
          }
          frame True {
            n101 = call "OUINON.vi"("errin"=w309, "image"="CONTEST") -> ("error out"=w308:errorcluster, "OUI/NON"=w307:bool)  [unwired: 8 in]
          }
        }
        n102 = local write "TOP"("Mesure de continuité" ("TOP")) -> ()
        n103 = case shown="Vrai" w282 {
          selector: w282 -> [w312 _]
          tunnel: w284 -> [w313 w321]
          tunnel: [w313 w317] -> w278
          tunnel: [w312 w319] -> w290
          tunnel: ["0" w314] -> w286
          tunnel: ["ERR" w314] -> w276
          frame False {
          }
          frame True {
            w320 = i16 2 ("largeur (-)")
            n104 = call "Impédance"("Enable"=TRUE, "error in (no error)"=w321) -> ("Conti"=w315:dbl, "error out"=w317:errorcluster)  [unwired: 15 in, 1 out]
            n105 = global read "OP500ZP_VGConf.vi" "Rmax"() -> (w316:dbl)
            n106 = Less Or Equal?(x=w315, y=w316) -> (x <= y?=w319:bool)
            n107 = Number To Fractional String(number=w315, width (-)=w320, precision (6)=w320) -> (F-format string=w314:string)  [unwired: 1 in]
          }
        }
        n108 = call "OUINON.vi"("errin"=w278, "image"="MSDOUT" ("IN")) -> ("error out"=w277:errorcluster)  [unwired: 8 in, 1 out]
        n109 = local read "Cluster"() -> (w288:T1)
        n110 = Concatenate Strings("Conti;" ("chaîne"), w276) -> (w301:string)
        n111 = Bundle By Name(cluster=w288, "Conti"=w286) -> (w287:T1)
        n112 = call "Log_basic.vi"("errin"=w299, "date?"=TRUE, "chaîne"=w301, "in"=w298) -> ("sortie d'erreur"=w296:errorcluster, "refnum en sortie"=w297:refnum<file>)  [unwired: 6 in]
        n113 = call "ZenPlusOP300_refaire.vi"("image"="Refaire", "refaire"=w291, "casOK"=OP500ZP_state."DTC", "errin"=w277, "test ok ?"=w290) -> ("errout"=w292:errorcluster, "Next"=w280:T4)  [unwired: 5 in]
        n114 = local write "Cluster"(w287) -> ()
      }
      frame "DTC" {
        # "Chercher moyen de simplifier"
        # "Vérification de l'absence de DTC dans FDT"
        n115 = call "OUINON.vi"("errin"=w328, "image"="DTC1" ("IN")) -> ("error out"=w345:errorcluster, "OUI/NON"=w346:bool)  [unwired: 8 in]
        n116 = case shown="Faux" w346 {
          tunnel: w345 -> [w366 w372]
          tunnel: [w366 w369] -> w327
          tunnel: [w365 w370] -> w326
          tunnel: [w365 w368] -> w322
          tunnel: [w365 w367] -> w323
          frame False {
            w365 = FALSE ("Aucun DTC")
          }
          frame True {
            n117 = call "Boîte de dialogue utilisateur"("Enable"=TRUE, "error in (no error)"=w372) -> ("Présence de DTC"=w367:bool, "Aucun DTC"=w368:bool, "OK"=w370:bool, "error out"=w369:errorcluster)  [unwired: 14 in]
            n118 = call "OUINON.vi"("image"="DTC2" ("IN")) -> ()  [unwired: 9 in, 2 out]
          }
        }
        n119 = And(x=w326, y=w322) -> (x .and. y?=w324:bool)
        n120 = case shown="Vrai" w324 {
          selector: w324 -> [_ w353]
          tunnel: [w348 w352] -> w325
          tunnel: w323 -> [w349 w354]
          frame False {
            n121 = case shown="Faux" w349 {
              tunnel: [FALSE FALSE] -> w348
              frame False {
              }
              frame True {
              }
            }
          }
          frame True {
            n122 = case shown="Vrai" w354 {
              tunnel: w353 -> [w355 _]
              tunnel: [w355 FALSE] -> w352
              frame False {
              }
              frame True {
              }
            }
          }
        }
        n123 = case shown="Vrai" w325 {
          selector: w325 -> [w358 w361]
          tunnel: w327 -> [w359 w364]
          tunnel: [w359 w362] -> w343
          tunnel: [w358 w361] -> w338
          tunnel: [";DTC DETECTE(S)" "NO DTC;"] -> w330
          frame False {
          }
          frame True {
            n124 = call "OUINON.vi"("errin"=w364, "image"="DTC3" ("IN")) -> ("error out"=w362:errorcluster)  [unwired: 8 in, 1 out]
          }
        }
        n125 = Concatenate Strings("DTC;" ("chaîne"), w330) -> (w337:string)
        n126 = call "Log_basic.vi"("errin"=w334, "date?"=TRUE, "chaîne"=w337, "in"=w332) -> ("sortie d'erreur"=w333:errorcluster, "refnum en sortie"=w331:refnum<file>)  [unwired: 6 in]
        n127 = call "ZenPlusOP300_refaire.vi"("image"="Refaire", "refaire"=w341, "casOK"=OP500ZP_state."Next", "errin"=w343, "test ok ?"=w338) -> ("errout"=w342:errorcluster, "Next"=w339:T4)  [unwired: 5 in]
      }
      frame "DataDyn" {
        w375 = OP500ZP_state."DataDyn"  # Énum
        w384 = enum16{"STR", "DBL", "U32"}."DBL" ("Énum")
        w387 = "Vpack" ("section")
        # "tension du pack en sortie"
        n128 = call <vilib>:"Application Directory.vi"() -> ("Application Directory"=w385:path)
        n129 = call "Read_Param.vi"("Énum"=w384, "errin"=w389, "pathin"=w385, "section"=w387, "key"="Min") -> ("error out"=w390:errorcluster, "dbl"=w382:dbl)  [unwired: 2 in, 3 out]
        n130 = call "Read_Param.vi"("Énum"=w384, "errin"=w390, "pathin"=w385, "section"=w387, "key"="Max") -> ("error out"=w388:errorcluster, "dbl"=w383:dbl)  [unwired: 2 in, 3 out]
        n131 = call "OUINON.vi"("errin"=w388, "image"="Vpack" ("IN")) -> ("error out"=w392:errorcluster, "OUI/NON"=w379:bool)  [unwired: 8 in]
        n132 = case shown="Vrai" w379 {
          selector: w379 -> [w399 _]
          tunnel: w392 -> [w401 w409]
          tunnel: [w401 w406] -> w393
          tunnel: ["ERR" w407] -> w377
          tunnel: [w399 w404] -> w378
          tunnel: w383 -> [_ w402]
          tunnel: w382 -> [_ w403]
          frame False {
          }
          frame True {
            w408 = i16 3 ("largeur (-)")
            n133 = call "Tension de l'étage bas"("error in (no error)"=w409) -> ("Vpack"=w405:dbl, "error out"=w406:errorcluster)  [unwired: 16 in, 1 out]
            n134 = In Range and Coerce(upper limit=w402, x=w405, lower limit=w403) -> (In Range?=w404:bool)  [unwired: 1 out]
            n135 = Number To Fractional String(number=w405, width (-)=w408, precision (6)=w408) -> (F-format string=w407:string)  [unwired: 1 in]
          }
        }
        n136 = Concatenate Strings("Vpack;" ("chaîne"), w377) -> (w380:string)
        n137 = call "Log_basic.vi"("errin"=w398, "chaîne"=w380, "in"=w397) -> ("sortie d'erreur"=w395:errorcluster, "refnum en sortie"=w396:refnum<file>)  [unwired: 7 in]
        n138 = call "OP500ZP_OuCrash.vi"("Booléen"=w378, "in"=w375) -> ("OUT"=w374:T4)  [unwired: 1 in]
      }
      frame "DataDyn2" {
        n139 = disable-structure shown="Désactivé" {
          disable-tunnel: [w458 _] -> w410
          disable-tunnel: w419 -> [w457 _]
          disable-tunnel: w418 -> [w456 _]
          disable-tunnel: w417 -> [w455 _]
          disable-tunnel: w415 -> [w454 _]
          disable-tunnel: [w453 _] -> w414
          disable-tunnel: [w452 _] -> w413
          disable-tunnel: [w451 _] -> w412
          disable-tunnel: w411 -> [w450 _]
          frame Disabled {
            w435 = OP500ZP_state."Demontage" ("Énum")
            n140 = property on="progression" class="Gliss (strict)"(error in=w450, "Visible"=TRUE, "Value"=u8 0 ("progression")) -> (error out=w440:errorcluster)  [unwired: 1 in, 1 out]
            n141 = local write "TOP"("Analyse 2 des CMU ..." ("TOP")) -> ()
            n142 = flat-sequence {
              tunnel: [w470] -> w423
              tunnel: [w469] -> w449
              tunnel: [w468] -> w448
              tunnel: [w467] -> w447
              tunnel: [w466] -> w446
              tunnel: [w465] -> w445
              tunnel: w440 -> [w464]
              frame #0 {
                n143 = call "SCAN CMU.vi"("errin"=w464, "Nb modules"=i16 16) -> ("errout"=w470:errorcluster, "# température + #tension OK?"=w465:bool, "Vmin"=w469:dbl, "Vmax"=w468:dbl, "Tmin"=w466:dbl, "Tmax"=w467:dbl)  [unwired: 4 out]
                n144 = call "FGV_Image.vi"("Énum"=FGV."SET", "IN"="DataDyn") -> ()  [unwired: 9 in, 1 out]
              }
            }
            n145 = global read "IS30%.vi" "VG IS30% ?"() -> (w421:bool)
            n146 = call "OP400ZP_Test_DataDyn.vi"("Tcell Min (°C)"=w446, "appdir"=w456, "is30%?"=w421, "MCU"=w445, "Tcell Max (°C)"=w447, "Température usine (°C)"=21.0, "errin"=w423, "testname"="Dyn2;", "Vcell Min (V)"=w449, "Vcell Max (V)"=w448) -> ("pass"=w422:bool, "datalog"=w460:string, "StrData"=w426:T7, "errout"=w424:errorcluster)  [unwired: 1 in, 1 out]
            n147 = Unbundle By Name(w426) -> ("Chaîne"=w431:string, "Chaîne"=w430:string, "Chaîne"=w429:string, "Chaîne"=w428:string, "Chaîne"=w427:string)
            n148 = call "Log_basic.vi"("errin"=w454, "date?"=TRUE, "chaîne"=w460, "in"=w455) -> ("sortie d'erreur"=w453:errorcluster, "refnum en sortie"=w452:refnum<file>)  [unwired: 6 in]
            n149 = local read "Cluster"() -> (w433:T1)
            n150 = Bundle By Name(cluster=w433, "2_TCellmin"=w431, "2_TCellmax"=w430, "2_VCellmin"=w429, "2_VCellmax"=w428, "2_Nbmodule"=w427) -> (w432:T1)
            n151 = call "ZenPlusOP300_refaire.vi"("image"="Refaire", "refaire"=w457, "Pédale"=FALSE, "errin"=w424, "test ok ?"=w422) -> ("errout"=w436:errorcluster, "Next"=w458:T4, "casOK"=w420:T4)  [unwired: 4 in]
            n152 = local write "Cluster"(w432) -> ()
            n153 = property on="progression" class="Gliss (strict)"(error in=w436, "Visible"=FALSE, "Value"=u8 0 ("progression")) -> (error out=w451:errorcluster)  [unwired: 1 in, 1 out]
          }
          frame Enabled {
          }
        }
      }
      frame "Crash" {
        # "\\\\forseepower.com\\fr\\040 Production\\FR7 - Poitiers\\06 Production\\05. Electronique\\Documents Control lib\\Archives\\ZEN PLUS"
        n154 = Close File(refnum=w499, error in=w498) -> (path=w483:path, error out=w491:errorcluster)
        n155 = call "FGV_Image.vi"("Énum"=FGV."SET", "IN"="TeamLeader") -> ()  [unwired: 9 in, 1 out]
        n156 = call "waitXms.vi"("attente (ms)"=u32 500, "errin"=w491) -> ("errout"=w484:errorcluster)  [unwired: 13 in]
        n157 = Read from Text File(file (use dialog)=w483, error in=w484) -> (text=w482:string, error out=w480:errorcluster)  [unwired: 2 in, 2 out]
        n158 = call "OP500ZP_SN_Reader.vi"("Fichier txt"=w482) -> ("SN"=w475:string)  [unwired: 10 in]
        n159 = local read "Cluster"() -> (w477:T1)
        n160 = Unbundle By Name(w477) -> ("PN"=w474:string)
        n161 = Concatenate Strings(w474, "-SN" ("chaîne"), w475) -> (w476:string)
        n162 = call "OP500ZP_NouveauDossier.vi"("entrée d'erreur (pas d'erreur)"=w480, "Nom du repertoire (PN SN)"=w476, "Network before adding a new folder"=path "D:/CODE/18 ZENX/OP500/Log et conf" ("chemin de la cible (utiliser une boîte de dialogue)")) -> ("sortie d'erreur"=w481:errorcluster, "Network after adding a new folder"=w478:path)  [unwired: 7 in]
        n163 = Copy ("Copier")(8:w481, 10:w478, 11:w483) -> (0:w490:errorcluster)  [unwired: 2 in, 2 out]
        n164 = call "PvgeneratorOP500.vi"("errin"=w490, "network"=w478, "path in"=w483) -> ("sortie d'erreur"=w494:errorcluster, "network out"=w493:path)  [unwired: 5 in, 2 out]
        n165 = Select ("Sélectionner")(t="1", s=FALSE ("sélecteur"), f="0" ("cas faux")) -> (s? t:f=w486:string)
        n166 = call "POP_GOOGLE.vi"("error in"=w494, "chemin"=w493) -> ("error out"=w471:errorcluster)  [unwired: 8 in, 1 out]
        n167 = local read "Cluster"() -> (w489:T1)
        n168 = Bundle By Name(cluster=w489, "Résultat final"=w486) -> ()  [unwired: 1 out]
        n169 = flat-sequence {
          tunnel: [TRUE] -> w500
          tunnel: w471 -> [_]
          frame #0 {
          }
        }
      }
      frame "Next" {
        w527 = OP500ZP_state."Null"  # Énum
        w528 = OP500ZP_state."Scan"  # Énum
        # "\\\\forseepower.com\\fr\\040 Production\\FR7 - Poitiers\\06 Production\\05. Electronique\\Documents Control lib\\Archives\\ZEN PLUS"
        n170 = Close File(refnum=w530, error in=w529) -> (path=w505:path, error out=w526:errorcluster)
        n171 = call "waitXms.vi"("attente (ms)"=u32 500, "errin"=w526) -> ("errout"=w517:errorcluster)  [unwired: 13 in]
        n172 = Read from Text File(file (use dialog)=w505, error in=w517) -> (text=w515:string, error out=w514:errorcluster)  [unwired: 2 in, 2 out]
        n173 = local read "Cluster"() -> (w510:T1)
        n174 = call "OP500ZP_SN_Reader.vi"("Fichier txt"=w515) -> ("SN"=w507:string)  [unwired: 10 in]
        n175 = call "OUINON.vi"("errin"=w532, "image"="Next" ("IN")) -> ("error out"=w504:errorcluster, "OUI/NON"=w531:bool)  [unwired: 8 in]
        n176 = Unbundle By Name(w510) -> ("PN"=w509:string)
        n177 = Concatenate Strings(w509, "-SN" ("chaîne"), w507) -> (w506:string)
        n178 = call "OP500ZP_NouveauDossier.vi"("entrée d'erreur (pas d'erreur)"=w514, "Nom du repertoire (PN SN)"=w506, "Network before adding a new folder"=path "\\\\forseepower.com\\fr/040 Production/FR7 - Poitiers/06 Production/05. Electronique/Documents Control lib/Archives/ZEN PLUS" ("chemin de la cible (utiliser une boîte de dialogue)")) -> ("sortie d'erreur"=w513:errorcluster, "Network after adding a new folder"=w511:path)  [unwired: 7 in]
        n179 = Copy ("Copier")(8:w513, 10:w511, 11:w505) -> (0:w516:errorcluster)  [unwired: 2 in, 2 out]
        n180 = call "PvgeneratorOP500.vi"("errin"=w516, "network"=w511, "path in"=w505) -> ("sortie d'erreur"=w524:errorcluster, "network out"=w523:path, "tout bon"=w521:bool)  [unwired: 5 in, 1 out]
        n181 = Select ("Sélectionner")(t="1", s=w521, f="0" ("cas faux")) -> (s? t:f=w518:string)
        n182 = local read "Cluster"() -> (w522:T1)
        n183 = Bundle By Name(cluster=w522, "Résultat final"=w518) -> ()  [unwired: 1 out]
        n184 = call "POP_GOOGLE.vi"("error in"=w524, "chemin"=w523) -> ("error out"=w502:errorcluster)  [unwired: 8 in, 1 out]
        n185 = Select(t=w528, s=w531, f=w527) -> (s? t:f=w503:T4)
      }
      frame "Comext" {
        n186 = disable-structure shown="Désactivé" {
          disable-tunnel: w544 -> [w558 _]
          disable-tunnel: w543 -> [w557 _]
          disable-tunnel: [w556 _] -> w542
          disable-tunnel: w541 -> [w555 _]
          disable-tunnel: [w554 _] -> w540
          disable-tunnel: w539 -> [w553 _]
          disable-tunnel: w538 -> [w551 _]
          disable-tunnel: [w549 _] -> w537
          disable-tunnel: w536 -> [w548 _]
          disable-tunnel: [w546 _] -> w535
          disable-tunnel: [w545 _] -> w534
          frame Disabled {
            n187 = call "OUINON.vi"("errin"=w551, "image"="Comext" ("IN")) -> ("error out"=w550:errorcluster, "OUI/NON"=w547:bool)  [unwired: 8 in]
            n188 = case shown="Vrai" w547 {
              tunnel: w558 -> [w563 w575]
              tunnel: w557 -> [w562 w574]
              tunnel: [w562 w573] -> w546
              tunnel: [w563 w572] -> w556
              tunnel: [OP500ZP_state."Crash" ("OUT") w571] -> w545
              tunnel: w555 -> [_ w570]
              tunnel: [w560 w569] -> w554
              tunnel: w553 -> [_ w568]
              tunnel: w550 -> [w560 w567]
              tunnel: [w561 w566] -> w549
              tunnel: w548 -> [w561 w566]
              frame False {
              }
              frame True {
                (unwired) "Comext;" ("testname")
                (unwired) OP500ZP_state."Demontage"  # Énum
                n189 = local read "PN"() -> (w586:string)
                n190 = call <vilib>:"Application Directory.vi"() -> ("Application Directory"=w588:path)
                n191 = call "Read_Param.vi"("Énum"=enum16{"STR", "DBL", "U32"}."U32", "errin"=w567, "pathin"=w588, "section"="DataDyn", "key"=w586) -> ("error out"=w581:errorcluster, "U32"=w584:u32)  [unwired: 2 in, 3 out]
                n192 = call "FGV_Image.vi"("Énum"=FGV."SET", "IN"="DataDyn") -> ()  [unwired: 9 in, 1 out]
                n193 = property on="progression" class="Gliss (strict)"(error in=w581, "Visible"=TRUE, "Value"=u8 0 ("progression")) -> (error out=w580:errorcluster)  [unwired: 1 in, 1 out]
                n194 = call "SCAN CMU.vi"("errin"=w580, "Nb modules"=w584) -> ("errout"=w598:errorcluster, "# température + #tension OK?"=w593:bool, "Vmin"=w597:dbl, "Vmax"=w596:dbl, "Tmin"=w594:dbl, "Tmax"=w595:dbl)  [unwired: 4 out]
                n195 = call "OP500ZP_Test_DataDyn.vi"("Vcell Max (V)"=w596, "MCU"=w593, "Vcell Min (V)"=w597, "appdir"=w568, "errin"=w598, "Température usine (°C)"=21.0, "Tcell Max (°C)"=w595, "Tcell Min (°C)"=w594) -> ("errout"=w592:errorcluster, "datalog"=w600:string, "pass"=w591:bool)  [unwired: 1 out]
                n196 = call "Log_basic.vi"("errin"=w575, "date?"=TRUE, "chaîne"=w600, "in"=w574) -> ("sortie d'erreur"=w572:errorcluster, "refnum en sortie"=w573:refnum<file>)  [unwired: 6 in]
                n197 = call "ZenPlusOP300_refaire.vi"("image"="Refaire", "refaire"=w570, "Pédale"=FALSE, "errin"=w592, "test ok ?"=w591) -> ("errout"=w576:errorcluster, "Next"=w571:T4)  [unwired: 5 in]
                n198 = property on="progression" class="Gliss (strict)"(error in=w576, "Visible"=FALSE, "Value"=u8 0 ("progression")) -> (error out=w569:errorcluster)  [unwired: 1 in, 1 out]
              }
            }
          }
          frame Enabled {
          }
        }
      }
      frame "MCU" {
        n199 = call "OP500ZP_FDT_V2.vi"("errin"=w617) -> ("errout"=w606:errorcluster, "Log"=w615:string)  [unwired: 8 in, 1 out]
        n200 = local write "TOP"("Mesure MCU" ("TOP")) -> ()
        n201 = call "Log_basic.vi"("errin"=w621, "date?"=TRUE, "chaîne"=w615, "in"=w620) -> ("sortie d'erreur"=w619:errorcluster, "refnum en sortie"=w618:refnum<file>)  [unwired: 6 in]
        n202 = global read "PackType.vi" "VG_PackType"() -> (w604:string)
        n203 = case shown="\"ZEN74\"" w604 {
          tunnel: [0 28 29 30 31 32] -> w607
          tunnel: [w660 w661 w663 w665 w667 w669] -> w605
          tunnel: w606 -> [w660 w661 w663 w665 w667 w669]
          frame "Faux", Default {
          }
          frame "ZEN74" {
          }
          frame "ZEN77" {
          }
          frame "ZEN79" {
          }
          frame "ZEN82" {
          }
          frame "ZEN84" {
          }
        }
        n204 = call "SCAN CMU.vi"("errin"=w605, "Nb modules"=w607) -> ("errout"=w608:errorcluster, "NbrTensions"=w602:i16, "NbrTemp"=w603:i16)  [unwired: 7 out]
        n205 = case shown="\"ZEN77\"" w604 {
          tunnel: w603 -> [_ w626 w637 w639 w646 w654]
          tunnel: w602 -> [_ w625 w634 w638 w645 w653]
          tunnel: [FALSE w624 w631 w640 w647 w652] -> w601
          frame "Faux", Default {
          }
          frame "ZEN74" {
            n206 = global read "OP500ZP_VGConf.vi" "ZEN74TENS"() -> (w629:dbl)
            n207 = global read "OP500ZP_VGConf.vi" "ZEN74TEMP"() -> (w630:dbl)
            n208 = Equal?(x=w626, y=w630) -> (x = y?=w627:bool)
            n209 = Equal?(x=w625, y=w629) -> (x = y?=w628:bool)
            n210 = And(x=w627, y=w628) -> (x .and. y?=w624:bool)
          }
          frame "ZEN77" {
            n211 = global read "OP500ZP_VGConf.vi" "ZEN77TENS"() -> (w635:dbl)
            n212 = global read "OP500ZP_VGConf.vi" "ZEN77TEMP"() -> (w636:dbl)
            n213 = Equal?(x=w637, y=w636) -> (x = y?=w632:bool)
            n214 = Equal?(x=w634, y=w635) -> (x = y?=w633:bool)
            n215 = And(x=w632, y=w633) -> (x .and. y?=w631:bool)
          }
          frame "ZEN79" {
            n216 = global read "OP500ZP_VGConf.vi" "ZEN79TENS"() -> (w643:dbl)
            n217 = global read "OP500ZP_VGConf.vi" "ZEN79TEMP"() -> (w644:dbl)
            n218 = Equal?(x=w639, y=w644) -> (x = y?=w641:bool)
            n219 = Equal?(x=w638, y=w643) -> (x = y?=w642:bool)
            n220 = And(x=w641, y=w642) -> (x .and. y?=w640:bool)
          }
          frame "ZEN82" {
            n221 = global read "OP500ZP_VGConf.vi" "ZEN82TENS"() -> (w650:dbl)
            n222 = global read "OP500ZP_VGConf.vi" "ZEN82TEMP"() -> (w651:dbl)
            n223 = Equal?(x=w646, y=w651) -> (x = y?=w648:bool)
            n224 = Equal?(x=w645, y=w650) -> (x = y?=w649:bool)
            n225 = And(x=w648, y=w649) -> (x .and. y?=w647:bool)
          }
          frame "ZEN84" {
            n226 = global read "OP500ZP_VGConf.vi" "ZEN84TENS"() -> (w657:dbl)
            n227 = global read "OP500ZP_VGConf.vi" "ZEN84TEMP"() -> (w658:dbl)
            n228 = Equal?(x=w654, y=w658) -> (x = y?=w655:bool)
            n229 = Equal?(x=w653, y=w657) -> (x = y?=w656:bool)
            n230 = And(x=w655, y=w656) -> (x .and. y?=w652:bool)
          }
        }
        n231 = call "ZenPlusOP300_refaire.vi"("image"="Refaire", "refaire"=w610, "casOK"=OP500ZP_state."OCVACIR", "errin"=w608, "test ok ?"=w601) -> ("errout"=w612:errorcluster, "Next"=w609:T4)  [unwired: 5 in]
      }
    }
    n232 = Wait (ms)(milliseconds to wait=u32 200 ("attente (ms)")) -> ()  [unwired: 1 out]
    n233 = case shown="Faux" w25 {
      selector: w25 -> [_ w671]
      frame False {
      }
      frame True {
        n234 = local write "STOP"(w671) -> ()
      }
    }
  }
  n235 = while {
    shift-right: [w680] -> _
    shift-left: errorcluster {"status"=FALSE, "code"=0, "source"=""} ("error out") -> [w677]
    stop <- w678 stop-if-true
    # "ici tu mets l'image à jour si besoin"
    n236 = Wait (ms)(milliseconds to wait=u32 100 ("attente (ms)")) -> ()  [unwired: 1 out]
    n237 = call "FGV_Image.vi"("Énum"=FGV."GET") -> ("OUT"=w673:string)  [unwired: 10 in]
    n238 = Not Equal?(x=w673, y="") -> (x != y?=w674:bool)
    n239 = case shown="Faux" w674 {
      tunnel: [w682 w687] -> w680
      tunnel: w677 -> [w682 w686]
      tunnel: w673 -> [_ w685]
      frame False {
      }
      frame True {
        n240 = call <vilib>:"Application Directory.vi"() -> ("Application Directory"=w690:path)
        n241 = Path To String(path=w690) -> (string=w691:string)
        n242 = Concatenate Strings(w691, "\\Image\\" ("chaîne"), w685, ".jpg" ("chaîne")) -> (w689:string)
        n243 = call "FGV_Image.vi"("Énum"=FGV."RAZ") -> ()  [unwired: 10 in, 1 out]
        n244 = String To Path(string=w689) -> (path=w688:path)
        n245 = call <vilib>:"Read JPEG File.vi"("error in (no error)"=w686, "path to JPEG file"=w688) -> ("error out"=w687:errorcluster, "image data"=w694:T8)  [unwired: 7 in, 1 out]
        n246 = call <vilib>:"Draw Flattened Pixmap.vi"("image data"=w694) -> ("new picture"=w683:picture)  [unwired: 8 in]
        n247 = local write "DRAW"(w683) -> ()
      }
    }
    n248 = global read "VG_progressBar.vi" "progression"() -> (→"progression":u8)
    n249 = local read "STOP"() -> (w679:bool)
    n250 = Or(x=w680, y=w679) -> (x .or. y?=w678:bool)
  }
  n251 = Merge Errors(w17, w16) -> (→"errout":errorcluster)
  n252 = disable-structure shown="Activé" {
    disable-tunnel: [w695 _] -> _
    frame Disabled {
      n253 = call "Data Dynamiques"() -> ("CMU OK"=w695:bool)  [unwired: 12 in, 7 out]
    }
    frame Enabled {
    }
  }
  "STOP" <- w14
